vi "RBVASS2mk2.vi"() -> ()   [LabVIEW 2021]
uses:
  <vilib>/vision/driver/IMAQdx.llb/IMAQdx Camera Control Mode.ctl
  <vilib>/vision/driver/IMAQdx.llb/IMAQdx Acquisition Mode.ctl
  <vilib>/vision/driver/IMAQdx.llb/IMAQdx Buffer Number Mode.ctl
  <vilib>/userDefined/High Color/IMAQdx.ctl
  <vilib>/myRIO/Instrument Drivers/Onboard IO/PWM/typedefs/PWM Reference.ctl
  <vilib>/myRIO/Common/Instrument Driver Framework/Utilities/typedefs/myRIO Generic Hardware Reference.ctl
  <vilib>/myRIO/Common/Instrument Driver Framework/Utilities/typedefs/Hardware Version Enum.ctl
  <vilib>/myRIO/Common/Instrument Driver Framework/Utilities/typedefs/myRIO v1.0 Reference.ctl
  <vilib>/myRIO/Common/Instrument Driver Framework/Utilities/typedefs/Generic FPGA Reference.ctl
  <vilib>/myRIO/Common/Instrument Driver Framework/myRIO v1.0/PWM/typedefs/PWM Channels Enum.ctl
  <vilib>/myRIO/Instrument Drivers/Onboard IO/PWM/typedefs/PWM Configuration.ctl
  <vilib>/userDefined/High Color/nirio_resource_hc.ctl
  <vilib>/myRIO/Instrument Drivers/Onboard IO/AI/typedefs/AI Reference.ctl
  <vilib>/myRIO/Common/Instrument Driver Framework/myRIO v1.0/AI/typedefs/AI Channels List.ctl
  <vilib>/myRIO/Common/Instrument Driver Framework/myRIO v1.0/AI/typedefs/AI Channels Enum.ctl
  <vilib>/myRIO/Common/Instrument Driver Framework/Utilities/typedefs/Analog Scaling Constants List.ctl
  <vilib>/myRIO/Common/Instrument Driver Framework/Utilities/typedefs/Analog Scaling Constants.ctl
  <vilib>/myRIO/Common/Instrument Driver Framework/myRIO v1.0/PWM/vis/myRIO v1.1 Open PWM.vi
  <vilib>/myRIO/Common/Instrument Driver Framework/myRIO v1.0/AI/vis/myRIO v1.1 Open AI.vi
  <vilib>/myRIO/Common/Instrument Driver Framework/Utilities/vis/Validate Channels.vi
  <vilib>/myRIO/Common/Instrument Driver Framework/myRIO v1.0/PWM/vis/myRIO v1.0 Reserve PWM.vi
  <vilib>/myRIO/Instrument Drivers/Onboard IO/PWM/vis/Set Duty Cycle and Frequency.vi
  <vilib>/myRIO/Common/Instrument Driver Framework/myRIO v1.0/PWM/vis/myRIO v1.0 Close PWM.vi
  <vilib>/myRIO/Common/Instrument Driver Framework/myRIO v1.0/AI/vis/myRIO v1.0 Reserve AI.vi
  <vilib>/myRIO/Common/Instrument Driver Framework/myRIO v1.0/AI/vis/myRIO v1.0 Close AI.vi
  <vilib>/myRIO/Common/Instrument Driver Framework/myRIO v1.0/PWM/vis/myRIO v1.0 Build MUX Configuration PWM.vi
  <vilib>/myRIO/Common/Instrument Driver Framework/myRIO v1.0/Resource Manager/vis/myRIO v1.0 Reserve Channel List.vi
  <vilib>/myRIO/Common/Instrument Driver Framework/myRIO v1.0/PWM/vis/myRIO v1.0 Unreserve PWM.vi
  <vilib>/myRIO/Common/Instrument Driver Framework/myRIO v1.0/AI/vis/myRIO v1.0 Build MUX Configuration AI.vi
  <vilib>/myRIO/Common/Instrument Driver Framework/myRIO v1.0/AI/vis/myRIO v1.0 Unreserve AI.vi
  <vilib>/myRIO/Common/Instrument Driver Framework/myRIO v1.0/Resource Manager/vis/myRIO v1.0 Create Configuration List.vi
  <vilib>/myRIO/Common/Instrument Driver Framework/myRIO v1.0/Resource Manager/vis/myRIO v1.0 Reserve Channel.vi
  <vilib>/myRIO/Common/Instrument Driver Framework/myRIO v1.0/Resource Manager/vis/myRIO v1.0 Unreserve Channel.vi
  <vilib>/myRIO/Common/Instrument Driver Framework/myRIO v1.0/Resource Manager/vis/myRIO v1.0 Unreserve Channel List.vi
  <vilib>/myRIO/Common/Instrument Driver Framework/myRIO v1.0/Resource Manager/vis/myRIO v1.0 Build Mutex Name.vi
  <vilib>/Utility/VariantDataType/GetNumericInfo.vi
  <vilib>/Utility/error.llb/Error Cluster From Error Code.vi
  <vilib>/myRIO/Common/Instrument Driver Framework/myRIO v1.0/myRIO v1.1 Open.vi
  <vilib>/myRIO/Common/Instrument Driver Framework/myRIO v1.0/AI/vis/myRIO v1.0 Get Scaling Constants AI.vi
  <vilib>/myRIO/Common/Instrument Driver Framework/Utilities/vis/IO Manager.vi
  <vilib>/myRIO/Common/Instrument Driver Framework/Utilities/vis/Configuration Manager.vi
  <vilib>/myRIO/Common/Instrument Driver Framework/myRIO v1.0/myRIO v1.0 Close.vi
  <vilib>/myRIO/Common/Instrument Driver Framework/myRIO v1.0/AI/vis/myRIO v1.0 Read AI.vi
  <vilib>/myRIO/Common/Instrument Driver Framework/myRIO v1.0/Resource Manager/vis/myRIO v1.0 Configure IO.vi
  <vilib>/myRIO/Common/Instrument Driver Framework/myRIO v1.0/PWM/vis/myRIO v1.0 Write PWM.vi
  <vilib>/myRIO/Common/Instrument Driver Framework/myRIO v1.0/PWM/vis/myRIO v1.0 Shutdown PWM.vi
  <vilib>/myRIO/Instrument Drivers/Onboard IO/AI/vis/myRIO AI Open.xnode
  <vilib>/myRIO/Instrument Drivers/Onboard IO/PWM/vis/myRIO PWM Open.xnode
  <vilib>/myRIO/Instrument Drivers/Onboard IO/AI/AI.lvlib
  <vilib>/vision/driver/NI_Vision_Acquisition_Software.lvlib
  <vilib>/vision/NI_Vision_Development_Module.lvlib
  <vilib>/myRIO/Instrument Drivers/Onboard IO/PWM/PWM.lvlib
panel:
  out "circles":i32
  in  "ROI Descriptor":T1 {"Contours"."Type" items=["No Selection", "Point", "Line", "Rectangle", "Oval", "Polygon", "Freehand Region", "Annulus", "Unused2", "Unused3", "Broken Line", "Freehand Line", "Rotated Rectangle"]}
  out "Image 2":T2(plugin-control)
  in  "error in 2":errorcluster
  in  "Settings":T3={"Objects"=0, "Threshold"=128, "Reject Border"=FALSE, "Fill Holes"=FALSE, "Min Object Size"=FALSE, "Min Size"=3, "Max Object Size"=FALSE, "Max Size"=100, "Show Search Area"=FALSE, "Show Center"=TRUE, "Show Bounding Box"=TRUE} {"Objects" items=["Bright Objects", "Dark Objects"]; "Threshold" min=1 max=999999999 step=1; "Max Size" min=1 max=999999999 step=1; "Min Size" min=1 max=999999999 step=1}
  in  "error in":errorcluster
  in  "stop":bool
  out "object":i32
  out "Colour Value":u32
  out "Color Box":u32(colorbox)
  in  "Knob":dbl(knob) scale=0.0..180.0
  out "error out":errorcluster
  out "Slide":dbl(slide) scale=0.0..10.0
  out "Numeric":i32
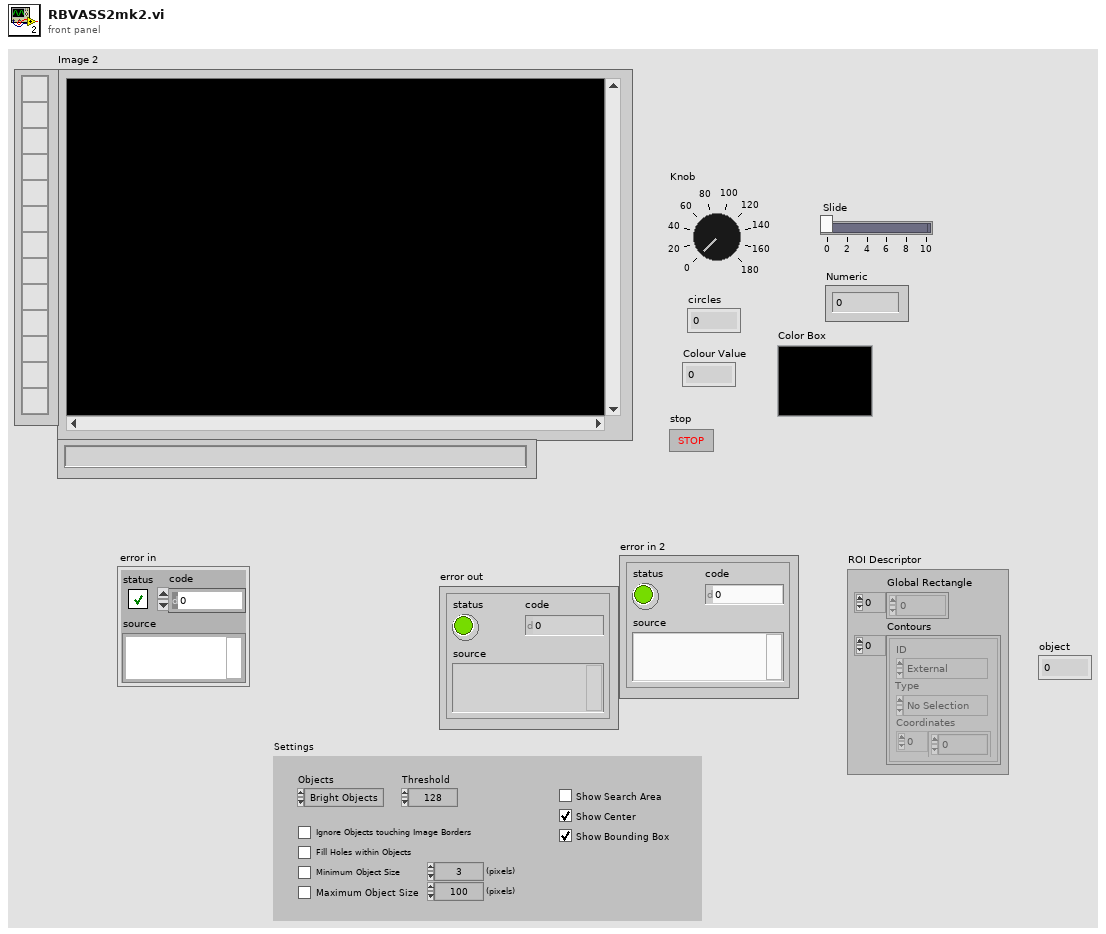
[diagram p1: front panel]
types:
  T1 = cluster{"Global Rectangle":i32[], "Contours":cluster{"ID":enum32{"External", "Internal"}, "Type":u32, "Coordinates":i32[]}[]}
  T2 = typedef "IMAQ Image.ctl" = refnum<image>
  T3 = cluster{"Objects":u16, "Threshold":i32, "Reject Border":bool, "Fill Holes":bool, "Min Object Size":bool, "Min Size":i32, "Max Object Size":bool, "Max Size":i32, "Show Search Area":bool, "Show Center":bool, "Show Bounding Box":bool}
  T4 = typedef "IMAQdx.ctl" = refnum<k21>
  T5 = typedef "NI_Vision_Acquisition_Software.lvlib/IMAQdx Buffer Number Mode.ctl" = enum32{"Next", "Last", "Buffer Number", "Every", "Last New"}
  T6 = typedef "NI_Vision_Acquisition_Software.lvlib/IMAQdx Acquisition Mode.ctl" = enum32{"One Shot", "Continuous"}
  T7 = typedef "NI_Vision_Acquisition_Software.lvlib/IMAQdx Camera Control Mode.ctl" = enum32{"Controller", "Listener"}
  T8 = typedef "PWM.lvlib/PWM Reference.ctl" = cluster{"myRIO Reference":T9, "PWM Channels Enum":T13, "PWM Configuration":T14}
  T9 = typedef "myRIO Generic Hardware Reference.ctl" = cluster{"myRIO Model":T10, "myRIO Hardware Reference":T11}
  T10 = typedef "Hardware Version Enum.ctl" = enum16{"Unknown", "myRIO-1900", "myRIO-1950", "roboRIO", "NI ELVIS RIO CM", "ELVIS III"}
  T11 = typedef "myRIO v1.0 Reference.ctl" = cluster{"Generic FPGA Reference":T12, "Allow multiple opens":bool}
  T12 = typedef "Generic FPGA Reference.ctl" = refnum<k20>
  T13 = typedef "PWM Channels Enum.ctl" = enum16{"Not Connected", "C/PWM0", "C/PWM1", "A/PWM0", "A/PWM1", "A/PWM2", "A/PWM3", "A/PWM4", "A/PWM5", "A/PWM6", "A/PWM7", "A/PWM8", "A/PWM9", "A/PWM10", "A/PWM11", "A/PWM12", "A/PWM13", "A/PWM14", "A/PWM15", "A/PWM16", "A/PWM17", "A/PWM18", "A/PWM19", "B/PWM0", "B/PWM1", "B/PWM2", "B/PWM3", "B/PWM4", "B/PWM5", "B/PWM6", "B/PWM7", "B/PWM8", "B/PWM9", "B/PWM10", "B/PWM11", "B/PWM12", "B/PWM13", "B/PWM14", "B/PWM15", "B/PWM16", "B/PWM17", "B/PWM18", "B/PWM19", "PWM/PWM0", "PWM/PWM1", "PWM/PWM2", "PWM/PWM3", "PWM/PWM4", "PWM/PWM5", "PWM/PWM6", "PWM/PWM7", "PWM/PWM8", "PWM/PWM9"}
  T14 = typedef "PWM.lvlib/PWM Configuration.ctl" = cluster{"Frequency":dbl, "Duty Cycle":dbl}
  T15 = typedef "AI.lvlib/AI Reference.ctl" = cluster{"myRIO Reference":T9, "AI Channels List":T16, "AI Scaling Constants List":T18}
  T16 = typedef "AI Channels List.ctl" = T17[]
  T17 = typedef "AI Channels Enum.ctl" = enum16{"Not Connected", "AudioIn/Left", "AudioIn/Right", "C/AI0", "C/AI1", "A/AI0", "A/AI1", "A/AI2", "A/AI3", "A/AI4", "A/AI5", "A/AI6", "A/AI7", "B/AI0", "B/AI1", "B/AI2", "B/AI3", "B/AI4", "B/AI5", "B/AI6", "B/AI7", "AI/AI0", "AI/AI1", "AI/AI2", "AI/AI3", "A/AI0 (DIFF)", "A/AI1 (DIFF)", "A/AI2 (DIFF)", "A/AI3 (DIFF)", "B/AI0 (DIFF)", "B/AI1 (DIFF)", "B/AI2 (DIFF)", "B/AI3 (DIFF)"}
  T18 = typedef "Analog Scaling Constants List.ctl" = T19[]
  T19 = typedef "Analog Scaling Constants.ctl" = cluster{"LSB Weight (Volts)":dbl, "Offset (Volts)":dbl, "Signed?":bool}
  T20 = typedef "Image Type" = u32
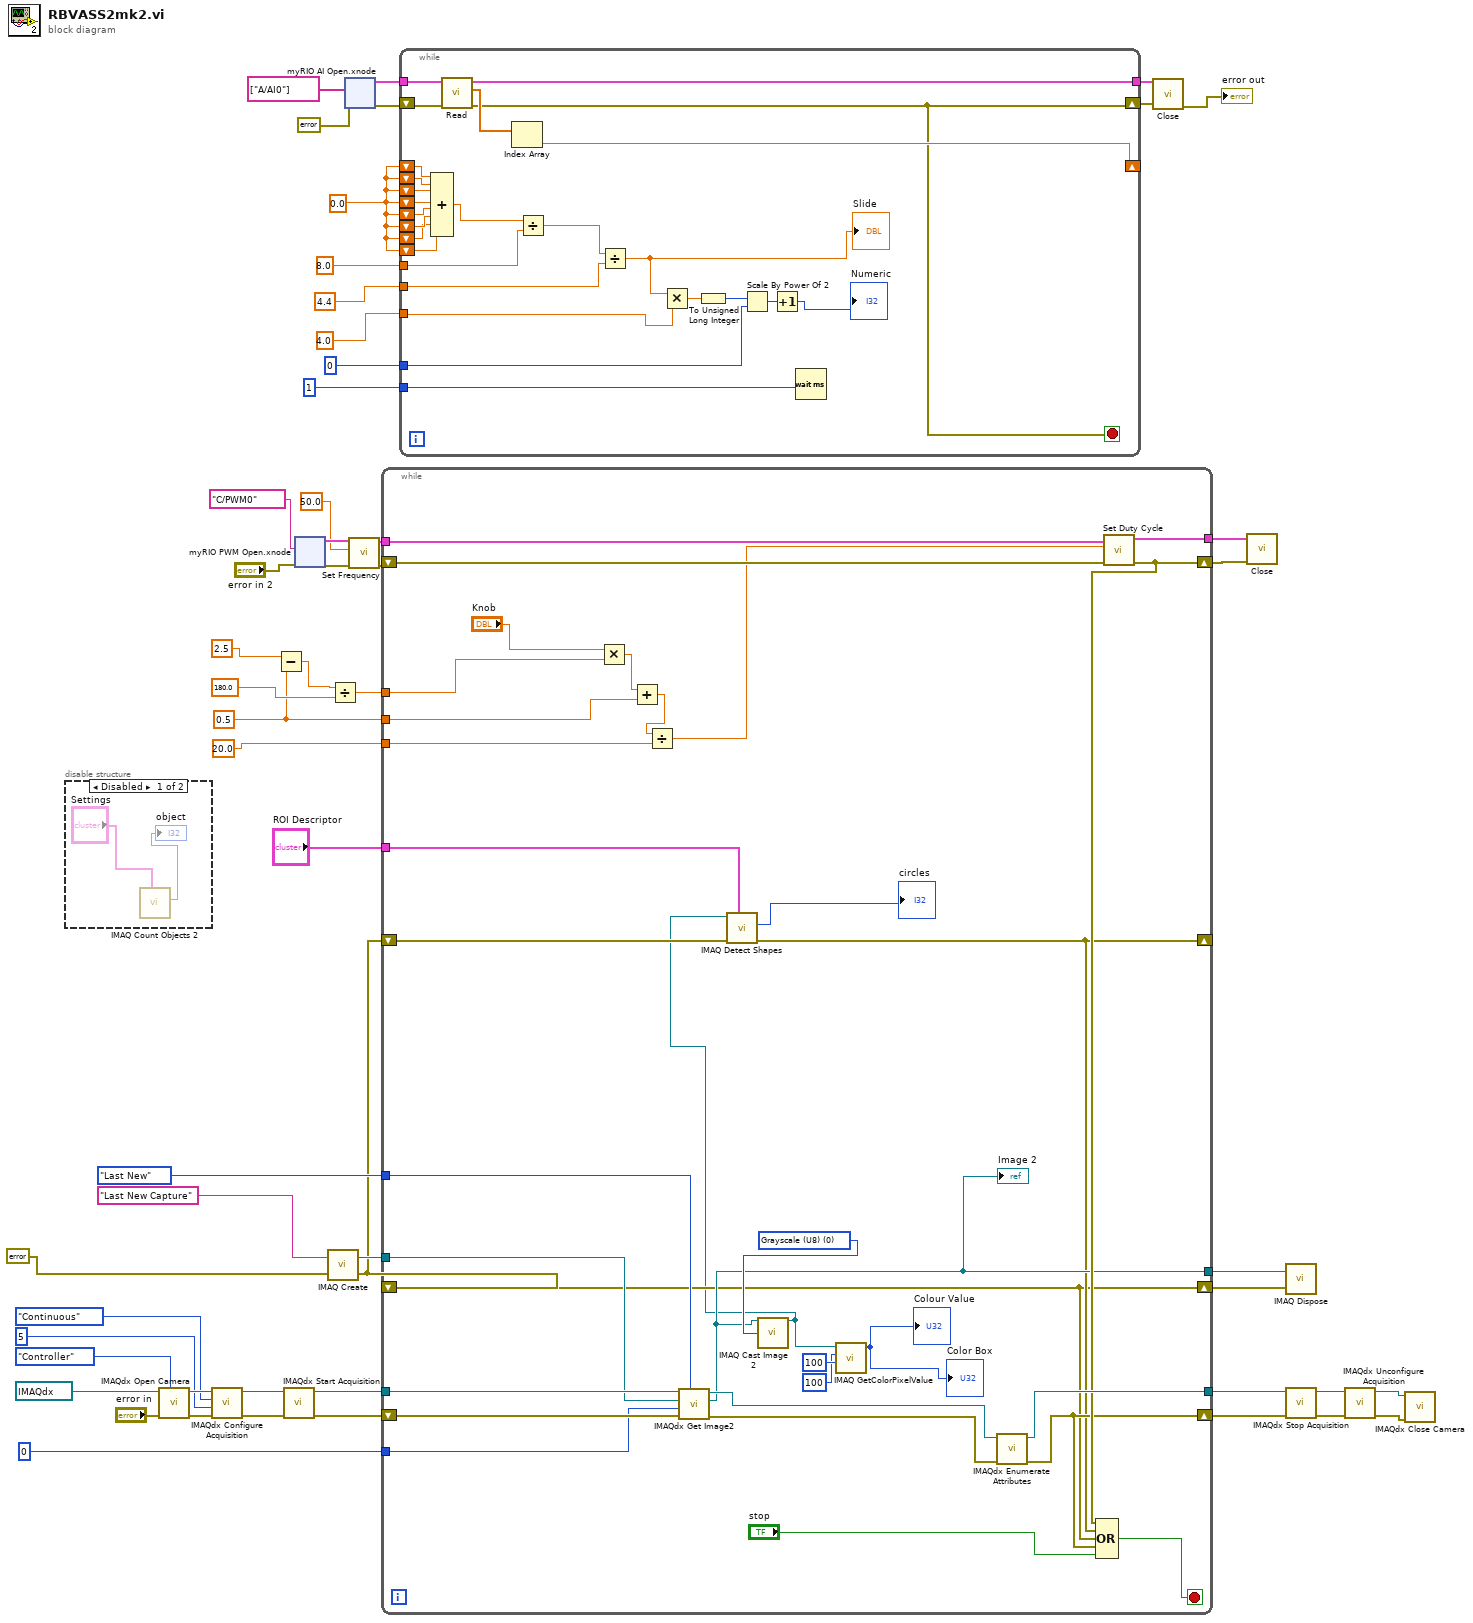
[diagram p0: block diagram]
diagram:
  w4 = 0.5
  w48 = 0.0
  n1 = disable-structure shown="Disabled" {
    frame Disabled {
      n2 = call "IMAQ Count Objects 2"("Settings"="Settings") -> ("Number of Objects"=→"object":i32)  [unwired: 6 in, 4 out]
    }
    frame Enabled {
    }
  }
  n3 = call <vilib>:"IMAQdx Open Camera.vi"("Camera Control Mode"=IMAQdx_Camera_Control_Mode."Controller", "error in"="error in", "Session In"=T4 "cam0") -> ("error out"=w34:errorcluster, "Session Out"=w35:T4)  [unwired: 7 in]
  n4 = call <vilib>:"IMAQdx Configure Acquisition.vi"("error in"=w34, "Number of Buffers"=u32 5, "Continuous?"=IMAQdx_Acquisition_Mode."Continuous", "Session In"=w35) -> ("error out"=w41:errorcluster, "Session Out"=w40:T4)  [unwired: 6 in]
  n5 = Subtract(x=2.5, y=w4) -> (x-y=w9:dbl)
  n6 = call <vilib>:"IMAQdx Start Acquisition.vi"("error in"=w41, "Session In"=w40) -> ("error out"=w28:errorcluster, "Session Out"=w29:T4)  [unwired: 8 in]
  n7 = xnode "myRIO PWM Open.xnode"("error in (no error)"="error in 2", "Channel Name"=tag "C/PWM0") -> ("error out"=w17:errorcluster, "PWM Ref Out"=w16:T8)  [unwired: 1 in]
  n8 = call "IMAQ Create"("Image Name"="Last New Capture", "error in (no error)"=errorcluster {"status"=FALSE, "code"=0, "source"=""} ("error in")) -> ("New Image"=w25:T2, "error out"=w1:errorcluster)  [unwired: 3 in]
  n9 = Divide(x=w9, y=180.0) -> (x/y=w5:dbl)
  n10 = xnode "myRIO AI Open.xnode"("error in (no error)"=errorcluster {"status"=FALSE, "code"=0, "source"=""}, "Channel Names"=tag[] ["A/AI0"]) -> ("error out"=w53:errorcluster, "AI Ref Out"=w54:T15)  [unwired: 1 in]
  n11 = call <vilib>:"Set Frequency.vi"("error in (no error)"=w17, "Frequency [Hz]"=50.0, "PWM Ref In"=w16) -> ("error out"=w13:errorcluster, "PWM Ref Out"=w11:T8)  [unwired: 6 in]
  n12 = while {
    tunnel: w29 -> [w89]
    shift-right: [w60] -> w23
    shift-left: w28 -> [w88]
    tunnel: w25 -> [w87]
    shift-right: [w58] -> w24
    shift-left: w1 -> [w58]
    tunnel: [w62] -> w22
    tunnel: [w86] -> w21
    tunnel: u32 0 ("Buffer Number In") -> [w84]
    shift-right: [w59] -> _
    shift-left: w1 -> [w65]
    tunnel: IMAQdx_Buffer_Number_Mode."Last New" ("Buffer Number Mode (Next)") -> [w83]
    shift-right: [w73] -> w12
    shift-left: w13 -> [w76]
    tunnel: w11 -> [w75]
    tunnel: [w74] -> w10
    tunnel: w4 -> [w69]
    tunnel: 20.0 -> [w68]
    tunnel: w5 -> [w67]
    tunnel: "ROI Descriptor" -> [w64]
    stop <- w82 stop-if-true
    w77 = T20 0 items=["Grayscale (U8)", "Grayscale (I16)", "Grayscale (SGL)", "Complex (CSG)", "RGB (U32)", "HSL (U32)", "RGB (U64)", "Grayscale (U16)"] ("Image Type")
    n13 = Multiply(x="Knob", y=w67) -> (x*y=w71:dbl)
    n14 = Add(x=w71, y=w69) -> (x+y=w70:dbl)
    n15 = Divide(x=w70, y=w68) -> (x/y=w66:dbl)
    n16 = call <vilib>:"IMAQdx Get Image2.vi"("Buffer Number Mode (Next)"=w83, "error in"=w88, "Buffer Number In"=w84, "Image In"=w87, "Session In"=w89) -> ("error out"=w85:errorcluster, "Image Out"=w62:T2, "Session Out"=w78:T4)  [unwired: 3 in, 1 out]
    "Image 2" <- w62
    n17 = call "IMAQ Cast Image 2"("Image Src"=w62, "Image Type"=w77) -> ("Image Dst Out"=w57:T2)  [unwired: 12 in, 1 out]
    n18 = call-poly "IMAQ Detect Shapes"("ROI Descriptor"=w64, "error in (no error)"=w65, "Image"=w57) -> ("error out"=w59:errorcluster, "Number of Matches Returned"=→"circles":i32)  [unwired: 6 in, 1 out]
    n19 = call "IMAQ GetColorPixelValue"("Y Coordinate"=100, "X Coordinate"=100, "Image"=w57) -> ("Pixel Value (U32)"=→"Colour Value" →"Color Box":u32)  [unwired: 1 in, 2 out]
    n20 = call <vilib>:"IMAQdx Enumerate Attributes.vi"("error in"=w85, "Session In"=w78) -> ("error out"=w60:errorcluster, "Session Out"=w86:T4)  [unwired: 7 in, 1 out]
    n21 = call <vilib>:"Set Duty Cycle.vi"("error in (no error)"=w76, "Duty Cycle"=w66, "PWM Ref In"=w75) -> ("error out"=w73:errorcluster, "PWM Ref Out"=w74:T8)  [unwired: 6 in]
    n22 = Compound Arithmetic op=OR(w73, w59, w58, w60, "stop") -> (w82:bool)
  }
  n23 = while {
    tunnel: w54 -> [w115]
    shift-right: [w99] -> w52
    shift-left: w53 -> [w114]
    tunnel: [w113] -> w51
    shift-right: [w111] -> _
    shift-left: w48 -> [w110]
    shift-left: w48 -> [w109]
    shift-left: w48 -> [w108]
    shift-left: w48 -> [w107]
    shift-left: w48 -> [w106]
    shift-left: w48 -> [w105]
    shift-left: w48 -> [w104]
    shift-left: w48 -> [w103]
    tunnel: 8.0 -> [w101]
    tunnel: u32 1 -> [w100]
    tunnel: 4.4 -> [w97]
    tunnel: 4.0 -> [w95]
    tunnel: 0 -> [w92]
    stop <- w99 stop-if-true
    n24 = Compound Arithmetic op=ADD(w110, w109, w108, w107, w106, w105, w104, w103) -> (w102:dbl)
    n25 = call <vilib>:"Read.vi"("error in (no error)"=w114, "AI Ref In"=w115) -> ("error out"=w99:errorcluster, "Values"=w112:dbl[], "AI Ref Out"=w113:T15)  [unwired: 7 in]
    n26 = Index Array(array=w112) -> (element=w111:dbl)  [unwired: 1 in]
    n27 = Divide(x=w102, y=w101) -> (x/y=w98:dbl)
    n28 = Divide(x=w98, y=w97) -> (x/y=w96:dbl)
    "Slide" <- w96
    n29 = Multiply(x=w96, y=w95) -> (x*y=w94:dbl)
    n30 = To Unsigned Long Integer(number=w94) -> (unsigned 32bit integer=w93:u32)
    n31 = Scale By Power Of 2(n=w93, x=w92) -> (x*2^n=w91:i32)
    n32 = Increment(x=w91) -> (x+1=→"Numeric":i32)
    n33 = Wait (ms)(milliseconds to wait=w100) -> ()  [unwired: 1 out]
  }
  n34 = call <vilib>:"Close.vi"("error in (no error)"=w52, "AI Ref In"=w51) -> ("error out"=→"error out":errorcluster)  [unwired: 9 in]
  n35 = call <vilib>:"Close.vi"("error in (no error)"=w12, "PWM Ref In"=w10) -> ()  [unwired: 9 in, 1 out]
  n36 = call "IMAQ Dispose"("Image"=w22, "error in (no error)"=w24) -> ()  [unwired: 4 in, 1 out]
  n37 = call <vilib>:"IMAQdx Stop Acquisition.vi"("error in"=w23, "Session In"=w21) -> ("error out"=w37:errorcluster, "Session Out"=w38:T4)  [unwired: 8 in]
  n38 = call <vilib>:"IMAQdx Unconfigure Acquisition.vi"("error in"=w37, "Session In"=w38) -> ("error out"=w36:errorcluster, "Session Out"=w39:T4)  [unwired: 8 in]
  n39 = call <vilib>:"IMAQdx Close Camera.vi"("error in"=w36, "Session In"=w39) -> ()  [unwired: 9 in, 1 out]
